vi "koniecgry_zapytanie.vi"(10 "Boolean":bool, 11 "Ring in":refnum<vi>) -> (3 "T button?":bool)   [LabVIEW 2016]
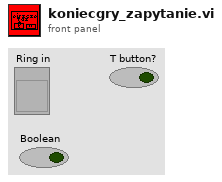
[diagram p1: front panel]
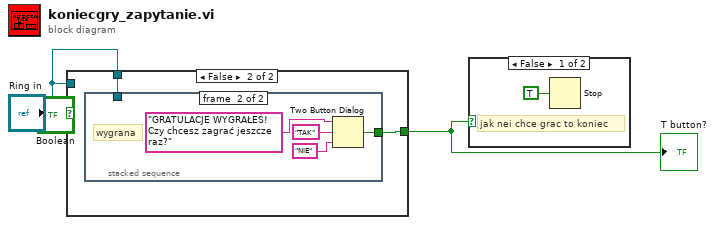
[diagram p0: block diagram]
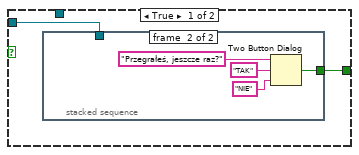
[diagram p2: hidden frame]
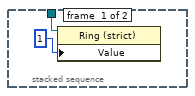
[diagram p3: hidden frame]
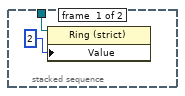
[diagram p4: hidden frame]
diagram:
  n1 = case shown="False" "Boolean" {
    tunnel: [w5 w13] -> w3
    tunnel: "Ring in" -> [w4 _]
    tunnel: "Ring in" -> [_ w12]
    frame True {
      n2 = stacked-sequence {
        tunnel: [_ w8] -> w5
        tunnel: w4 -> [w6 _]
        frame #0 {
          n3 = property class="Ring (strict)"(reference=w6, "Value"=u16 1 ("Ring")) -> ()  [unwired: 1 in, 2 out]
        }
        frame #1 {
          n4 = Two Button Dialog(message="Przegrałeś, jeszcze raz?", 1:"NIE" ("button name (\"OK\")"), 2:"TAK" ("button name (\"OK\")")) -> (T button?=w8:bool)
        }
      }
    }
    frame False {
      n5 = stacked-sequence {
        tunnel: [_ w18] -> w13
        tunnel: w12 -> [w14 _]
        frame #0 {
          n6 = property class="Ring (strict)"(reference=w14, "Value"=u16 2 ("Ring")) -> ()  [unwired: 1 in, 2 out]
        }
        frame #1 {
          # "wygrana"
          n7 = Two Button Dialog(message="GRATULACJE WYGRAŁEŚ! Czy chcesz zagrać jeszcze raz?", 1:"NIE" ("button name (\"OK\")"), 2:"TAK" ("button name (\"OK\")")) -> (T button?=w18:bool)
        }
      }
    }
  }
  "T button?" <- w3
  n8 = case shown="False" w3 {
    frame False {
      # "jak nei chce grac to koniec"
      n9 = Stop(stop? (T)=TRUE) -> ()
    }
    frame True {
    }
  }
